vi "Motor Controller Datastream (get N samples) with Rendezvous.vi"(8 "N samples":i32, 9 "Set data rate?":bool, 10 "Data rate (Hz)":u8(ring)=14 items=["1", "2", "4", "5", "8", "10", "16", "20", "25", "32", "40", "50", "64", "80", "100", "125", "160", "200", "250", "320", "400", "500", "625", "800", "1000"], 11 "COM port":refnum<visa-resource-name>) -> (0 "Error out":errorcluster, 1 "Chk err":u32, 2 "Frm err":u32, 3 "Data cluster array":T1[](array[typedef]))   [LabVIEW 2020]
uses:
  ctls/CTRL_Data_Out.ctl
  ctls/CTRL_Cmd.ctl
  Anemometry/Anemometry Sub Vis/Globals/Meas_global.vi
panel:
  in  "Stop":bool
  out "Datastream":T2(graph)
  # "RPM (/min)"
  # "I_m (A)"
  # "Photo (V)"
  # "Duty ()"
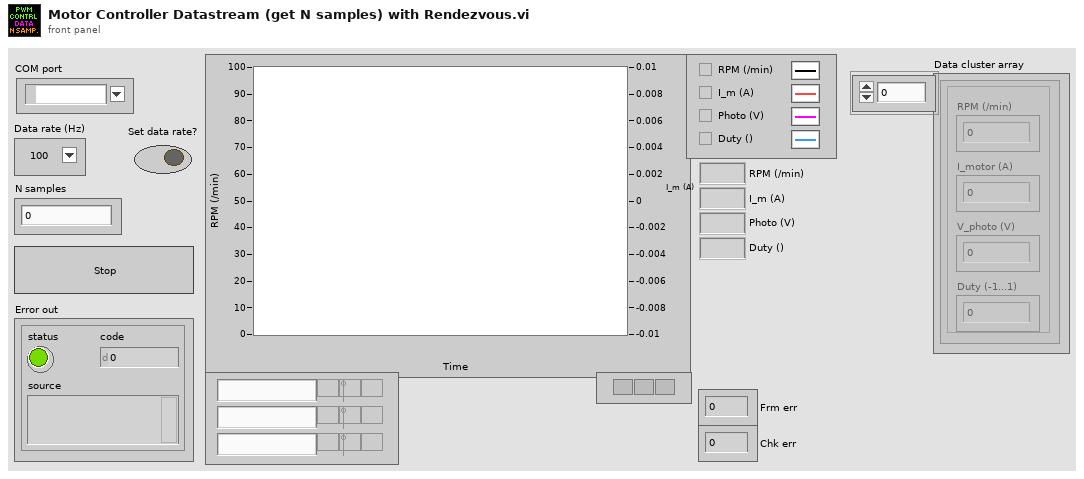
[diagram p1: front panel]
types:
  T1 = typedef "CTRL_Data_Out.ctl" = cluster{"RPM (/min)":sgl, "I_motor (A)":sgl, "V_photo (V)":sgl, "Duty (-1...1)":sgl}
  T2 = cluster{"RPM (/min)":sgl, "I_motor (A)":sgl, "V_photo (V)":sgl, "Duty (-1...1)":sgl}
  T3 = cluster{"RPM (/min)":sgl, "I_motor (A)":sgl, "V_photo (V)":sgl, "Duty (-1...1)":sgl}[]
  T4 = typedef "CTRL_Cmd.ctl" = string
  T5 = typedef "Rendezvous RefNum" = refnum<k1>
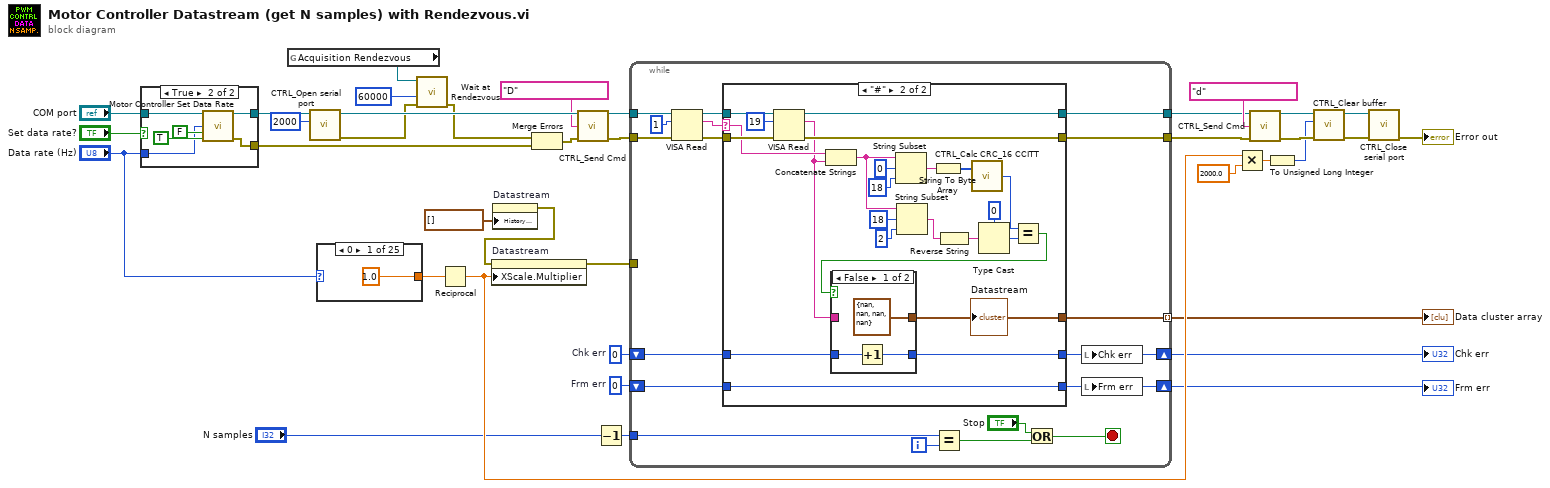
[diagram p0: block diagram]
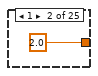
[diagram p2: hidden frame]
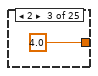
[diagram p3: hidden frame]
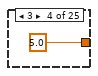
[diagram p4: hidden frame]
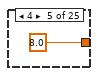
[diagram p5: hidden frame]
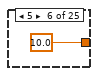
[diagram p6: hidden frame]
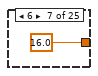
[diagram p7: hidden frame]
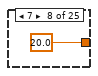
[diagram p8: hidden frame]
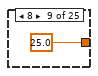
[diagram p9: hidden frame]
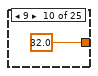
[diagram p10: hidden frame]
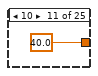
[diagram p11: hidden frame]
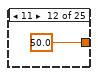
[diagram p12: hidden frame]
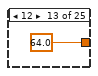
[diagram p13: hidden frame]
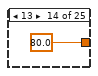
[diagram p14: hidden frame]
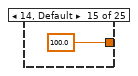
[diagram p15: hidden frame]
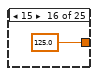
[diagram p16: hidden frame]
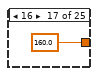
[diagram p17: hidden frame]
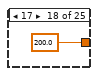
[diagram p18: hidden frame]
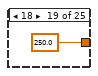
[diagram p19: hidden frame]
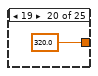
[diagram p20: hidden frame]
diagram:
  w13 = u32 0  # Chk err
  w14 = u32 0  # Frm err
  n1 = case shown="True" "Set data rate?" {
    tunnel: "COM port" -> [w40 w46]
    tunnel: [w40 w45] -> w18
    tunnel: [errorcluster {"status"=FALSE, "code"=0, "source"=""} ("Error out") w44] -> w16
    tunnel: "Data rate (Hz)" -> [_ w41]
    frame False {
    }
    frame True {
      n2 = call "Motor Controller Set Data Rate.vi"("COM port"=w46, "Data rate (Hz)"=w41, "Set as power-on default"=FALSE, "Close port after action"=TRUE) -> ("COM port out"=w45:refnum<visa-resource-name>, "Error out"=w44:errorcluster)  [unwired: 10 in]
    }
  }
  n3 = global read "Meas_global.vi" "Acquisition Rendezvous"() -> (w1:T5)
  n4 = call "CTRL_Open serial port.vi"("timeout (ms)"=u32 2000, "VISA resource name"=w18) -> ("Error out"=w4:errorcluster, "VISA resource name out"=w22:refnum<visa-resource-name>)  [unwired: 8 in]
  n5 = case shown="0" "Data rate (Hz)" {
    tunnel: [1.0 2.0 4.0 5.0 8.0 10.0 16.0 20.0 25.0 32.0 40.0 50.0 64.0 80.0 100.0 125.0 160.0 200.0 250.0 320.0 400.0 500.0 625.0 800.0 1000.0] -> w6
    frame 0 {
    }
    frame 1 {
    }
    frame 2 {
    }
    frame 3 {
    }
    frame 4 {
    }
    frame 5 {
    }
    frame 6 {
    }
    frame 7 {
    }
    frame 8 {
    }
    frame 9 {
    }
    frame 10 {
    }
    frame 11 {
    }
    frame 12 {
    }
    frame 13 {
    }
    frame 14, Default {
    }
    frame 15 {
    }
    frame 16 {
    }
    frame 17 {
    }
    frame 18 {
    }
    frame 19 {
    }
    frame 20 {
    }
    frame 21 {
    }
    frame 22 {
    }
    frame 23 {
    }
    frame 24 {
    }
  }
  n6 = call <vilib>:"Wait at Rendezvous.vi"("error in (no error)"=w4, "ms timeout (-1)"=60000, "rendezvous"=w1) -> ("error out"=w3:errorcluster)  [unwired: 2 in, 2 out]
  n7 = Reciprocal(x=w6) -> (1/x=w15:dbl)
  n8 = property on="Datastream" class="WFChart (strict)"("History Data"=T3 []) -> (error out=w34:errorcluster)  [unwired: 2 in, 1 out]
  n9 = property on="Datastream" class="WFChart (strict)"(error in=w34, "XScale.Multiplier"=w15) -> (error out=w25:errorcluster)  [unwired: 1 in, 1 out]
  n10 = Merge Errors(w3, w16) -> (w17:errorcluster)
  n11 = call "CTRL_Send Cmd.vi"("Port"=w22, "Cmd"=T4 "D" ("Command"), "Error In"=w17) -> ("Port out"=w23:refnum<visa-resource-name>, "Error Out"=w24:errorcluster)  [unwired: 11 in]
  n12 = Decrement(x="N samples") -> (x-1=w9:i32)
  n13 = while {
    tunnel: w23 -> [w89]
    tunnel: w24 -> [w88]
    tunnel: [w83] -> w31
    tunnel: [w82] -> w32
    tunnel: w25 -> [_]
    shift-right: [w72] -> w7
    shift-left: w14 -> [w81]
    shift-right: [w73] -> w8
    shift-left: w13 -> [w80]
    tunnel: [w79] -> w11 mode=indexing
    tunnel: w9 -> [w78]
    i -> [w76]
    stop <- w77 stop-if-true
    n14 = VISA Read(VISA resource name=w89, byte count=u32 1, error in (no error)=w88) -> (VISA resource name out=w85:refnum<visa-resource-name>, read buffer=w84:string, error out=w86:errorcluster)  [unwired: 1 out]
    n15 = case shown="\"#\"" w84 {
      selector: w84 -> [_ w114]
      tunnel: w86 -> [w95 w118]
      tunnel: w85 -> [w94 w119]
      tunnel: [w95 w116] -> w83
      tunnel: [w94 w115] -> w82
      tunnel: [w93 w99] -> w72
      tunnel: w81 -> [w92 w99]
      tunnel: [w91 w96] -> w73
      tunnel: w80 -> [w91 w98]
      tunnel: [T1 {"RPM (/min)"=nan, "I_motor (A)"=nan, "V_photo (V)"=nan, "Duty (-1...1)"=nan} ("Data") w97] -> w79
      frame Default {
        n16 = Increment(x=w92) -> (x+1=w93:u32)
      }
      frame "#" {
        n17 = VISA Read(VISA resource name=w119, byte count=u32 19, error in (no error)=w118) -> (VISA resource name out=w115:refnum<visa-resource-name>, read buffer=w113:string, error out=w116:errorcluster)  [unwired: 1 out]
        n18 = Concatenate Strings(w114, w113) -> (w101:string)
        n19 = String Subset(string=w101, offset (0)=0, length (rest)=18 ("length (rest)")) -> (substring=w100:string)
        n20 = String Subset(string=w101, offset (0)=18, length (rest)=2 ("length (rest)")) -> (substring=w109:string)
        n21 = String To Byte Array(string=w100) -> (unsigned byte array=w112:u8[])
        n22 = Reverse String(1:w109) -> (0:w107:string)
        n23 = call "CTRL_Calc CRC_16 CCITT.vi"("Data bytes"=w112) -> ("CRC_16-CCITT"=w106:u16)  [unwired: 1 in]
        n24 = Type Cast(type=u16 0 ("length (rest)"), x=w107) -> (*(type *) &x=w105:u16)
        n25 = Equal?(x=w106, y=w105) -> (x = y?=w104:bool)
        n26 = case shown="False" w104 {
          tunnel: w113 -> [_ w125]
          tunnel: [T1 {"RPM (/min)"=nan, "I_motor (A)"=nan, "V_photo (V)"=nan, "Duty (-1...1)"=nan} ("Data") w124] -> w97
          tunnel: [w122 w123] -> w96
          tunnel: w98 -> [w121 w123]
          frame False {
            n27 = Increment(x=w121) -> (x+1=w122:u32)
          }
          frame True {
            n28 = call "CTRL_Convert serial string to Eng vals.vi"("Serial buffer string (excluding FrameChar)"=w125) -> ("Data"=w124:T1)
          }
        }
        "Datastream" <- w97
      }
    }
    n29 = Equal?(x=w78, y=w76) -> (x = y?=w75:bool)
    n30 = Or(x="Stop", y=w75) -> (x .or. y?=w77:bool)
    n31 = local write "Chk err"(w73) -> ()
    n32 = local write "Frm err"(w72) -> ()
  }
  "Data cluster array" <- w11
  "Chk err" <- w8
  "Frm err" <- w7
  n33 = Multiply(x=w15, y=2000.0) -> (x*y=w28:dbl)
  n34 = call "CTRL_Send Cmd.vi"("Port"=w32, "Cmd"=T4 "d" ("Command"), "Error In"=w31) -> ("Port out"=w30:refnum<visa-resource-name>, "Error Out"=w29:errorcluster)  [unwired: 11 in]
  n35 = To Unsigned Long Integer(number=w28) -> (unsigned 32bit integer=w26:u32)
  n36 = call "CTRL_Clear buffer.vi"("Error in"=w29, "dt for timeout (ms)"=w26, "VISA resource name in"=w30) -> ("Error out"=w36:errorcluster, "VISA resource name out"=w37:refnum<visa-resource-name>)  [unwired: 3 in]
  n37 = call "CTRL_Close serial port.vi"("Error in"=w36, "VISA resource name"=w37) -> ("Error out"=→"Error out":errorcluster)  [unwired: 9 in]
